vi "LSX Move Ex.vi"(0 "lLSID":i32, 1 "dR":dbl, 2 "bWait":i32, 5 "dX":dbl, 7 "dY":dbl, 9 "dZ":dbl, 11 "error in (no error)":errorcluster, 12 "bRelative":i32, 13 "lAxisCount":i32) -> (4 "function return":i32, 15 "error out":errorcluster)   [LabVIEW 2018, in "Tango.lvlib"]
doc: "TANGOAPI int TANGOCALL LSX_MoveEx (int lLSID, double dX, double dY, double dZ, double dR, BOOL bRelative, BOOL bWait, int lAxisCount);"
uses:
  <userlib>/Tango/Tango.lvlib
  <userlib>/Tango/Tango_DLL.dll
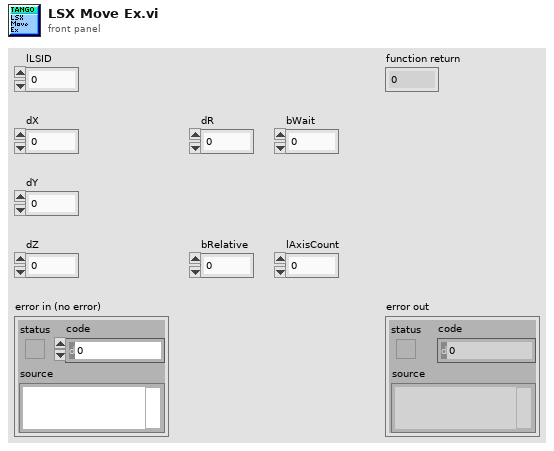
[diagram p1: front panel]
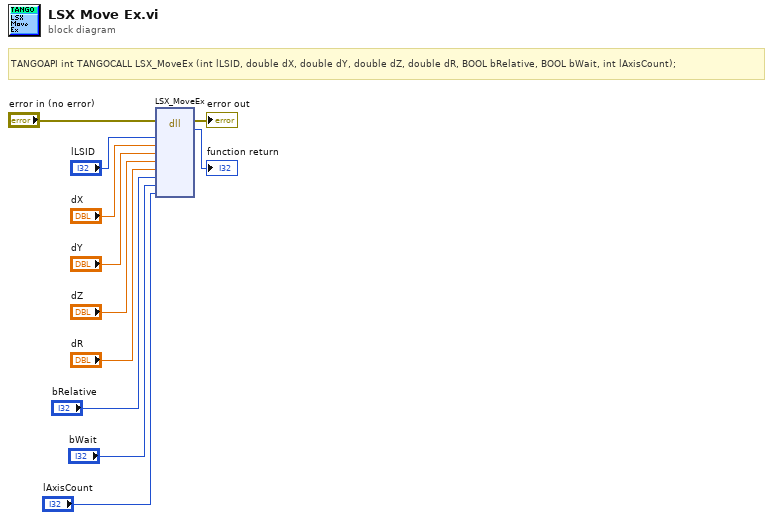
[diagram p0: block diagram]
diagram:
  # "TANGOAPI int TANGOCALL LSX_MoveEx (int lLSID, double dX, double dY, double dZ, double dR, BOOL bRelative, BOOL bWait, int lAxisCount);"
  n1 = dll-call lib="C:/Program Files (x86)/National Instruments/LabVIEW 2018/user.lib/Tango/Tango_DLL.*" fn="LSX_MoveEx"(error in="error in (no error)", "lLSID"="lLSID", "dX"="dX", "dY"="dY", "dZ"="dZ", "dR"="dR", "bRelative"="bRelative", "bWait"="bWait", "lAxisCount"="lAxisCount") -> (error out=→"error out":errorcluster, →"function return":i32)  [unwired: 10 in, 1 out]
